vi "SeqMgr.Sequence, Parse Line.vi"(6 "Levels":cluster{"If":i32, "For":i32, "While":i32}, 8 "error in":errorcluster, 10 "LineCnt":i32, 11 "Line":string) -> (0 "error out":errorcluster, 1 "Comment":string, 2 "Is Comment":bool, 3 "Step":string[](array[string]), 4 "Levels Out":cluster{"If":i32, "For":i32, "While":i32})   [LabVIEW 2024, in "EQMF.lvlib" / "SeqMgr.lvlib"]
uses:
  SeqMgr.lvlib
  <vilib>/Utility/error.llb/Trim Whitespace One-Sided.vi
  Strings/String Utils.lvlib
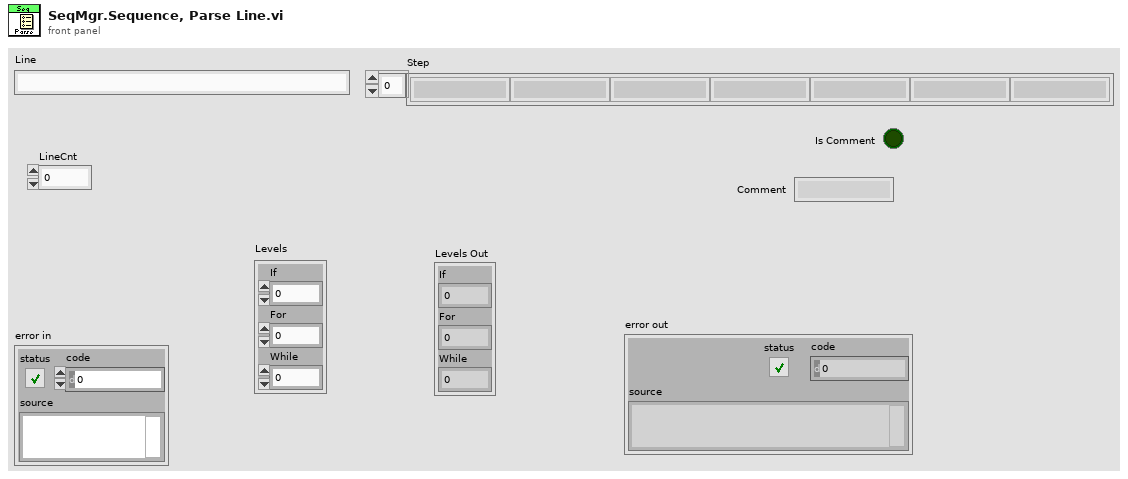
[diagram p1: front panel]
types:
  T1 = cluster{"Line":string, "Step":string[], "\nLevels":cluster{"If":i32, "For":i32, "While":i32}}
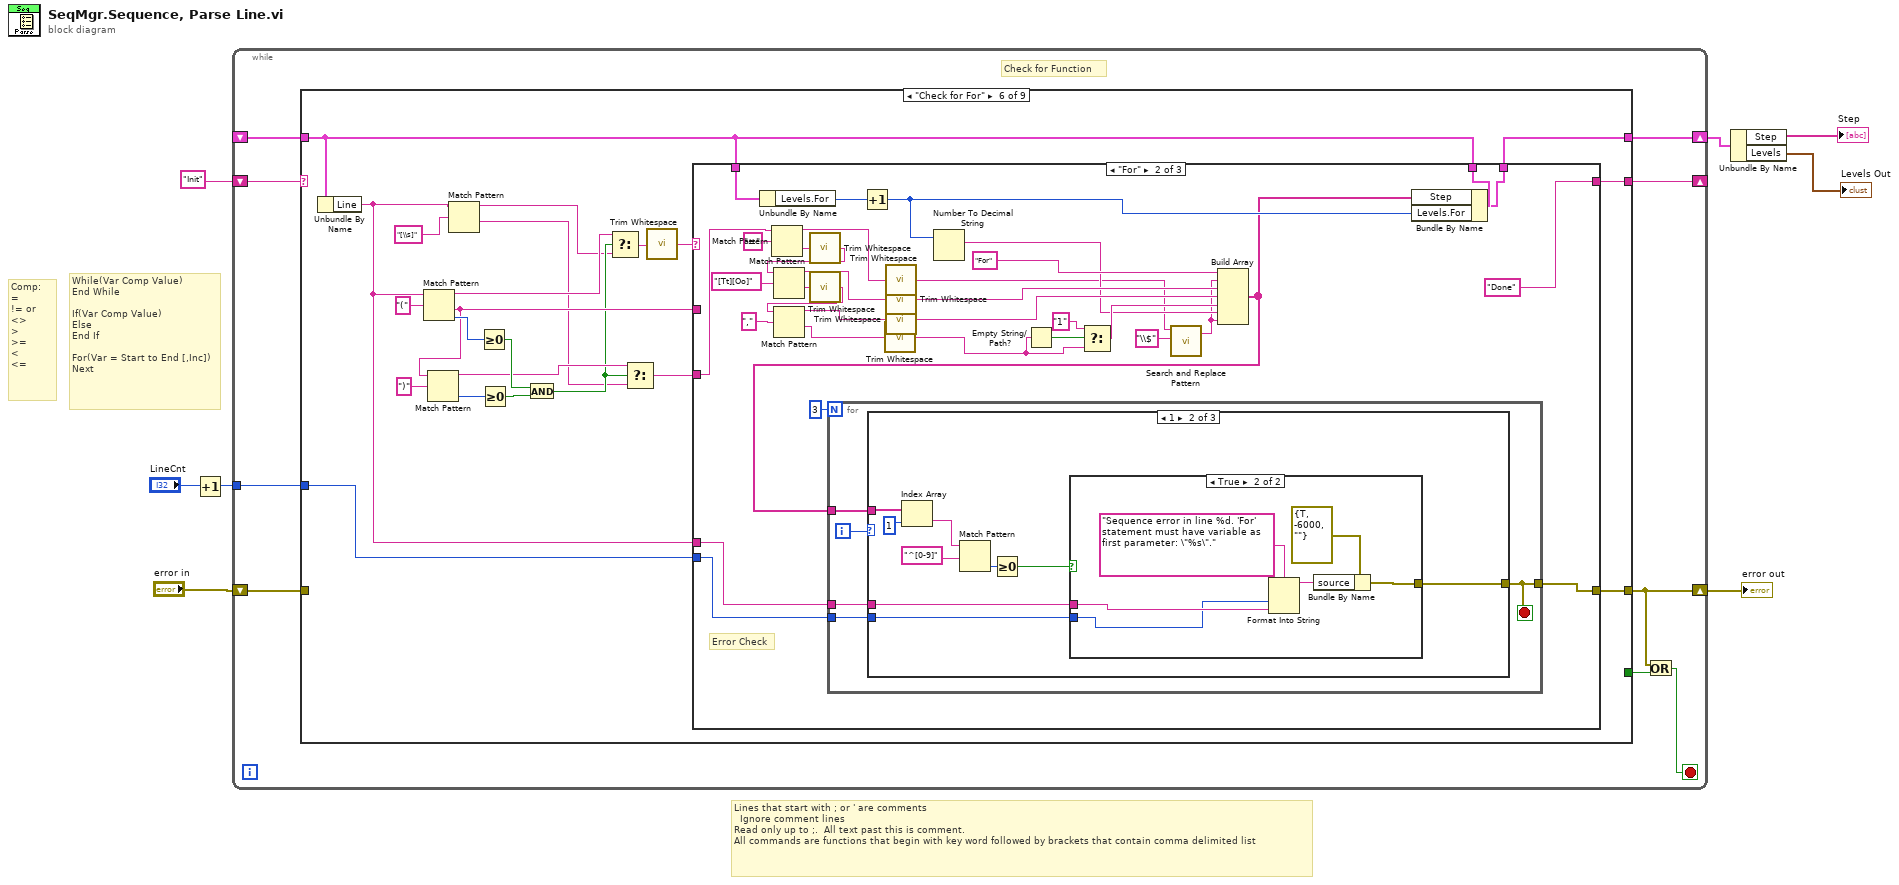
[diagram p0: block diagram]
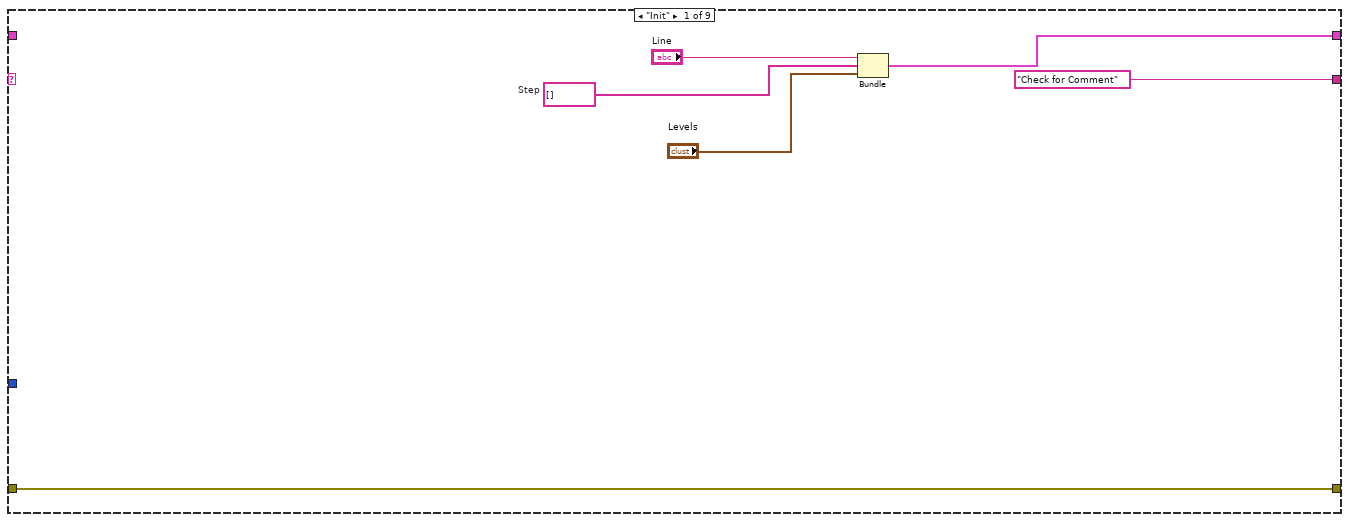
[diagram p2: hidden frame]
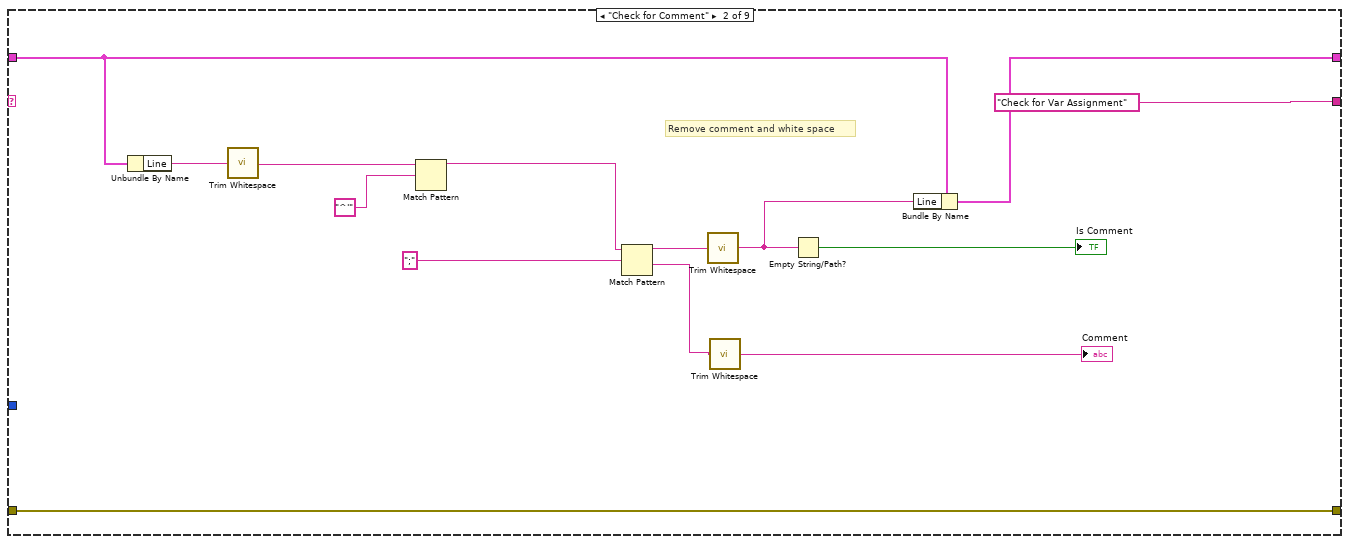
[diagram p3: hidden frame]
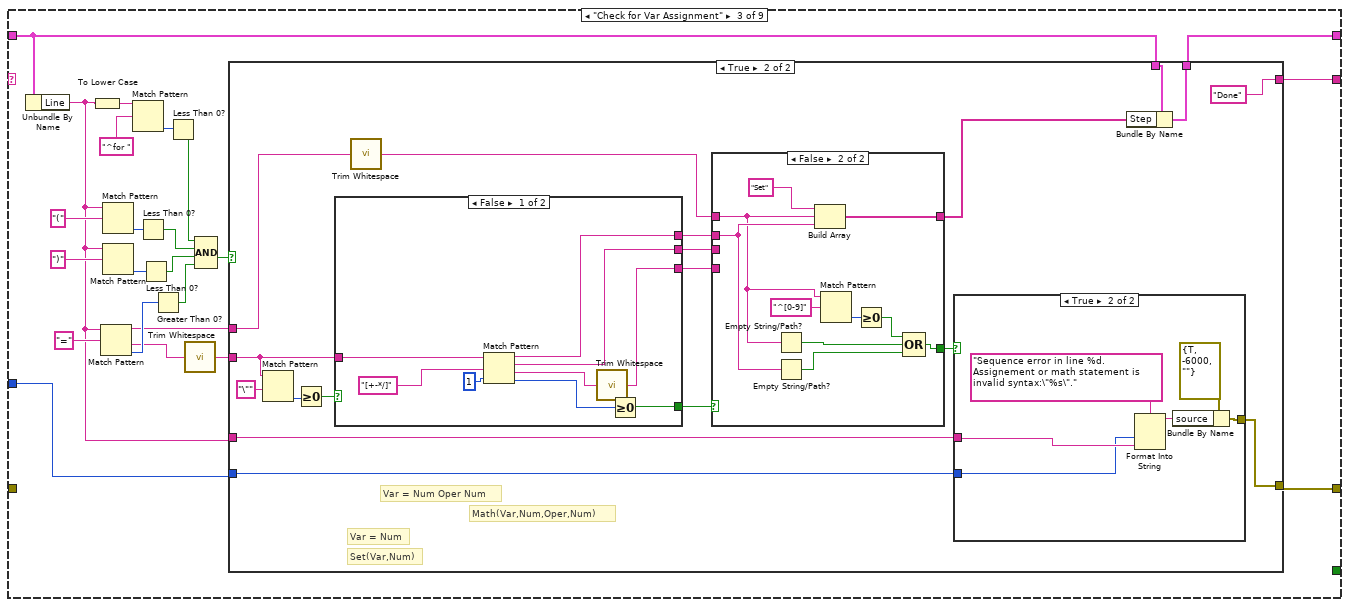
[diagram p4: hidden frame]
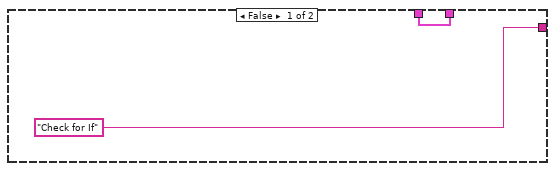
[diagram p5: hidden frame]
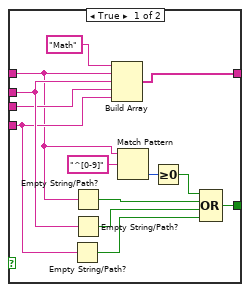
[diagram p7: hidden frame]
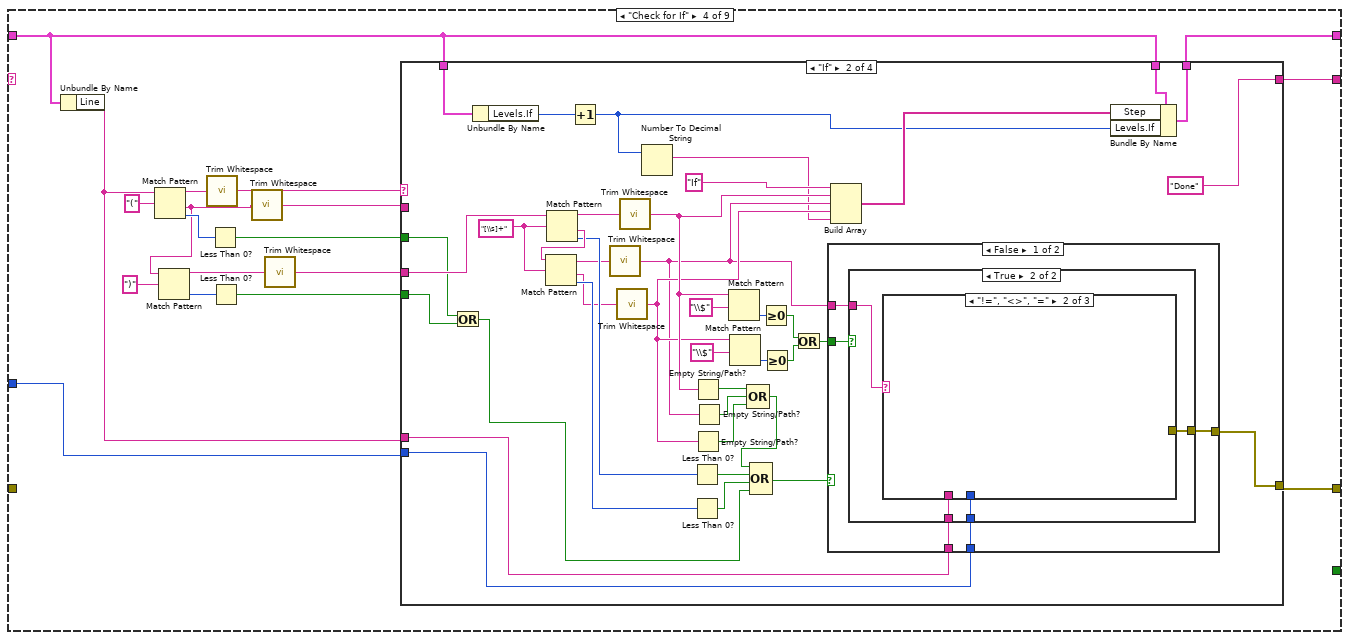
[diagram p9: hidden frame]
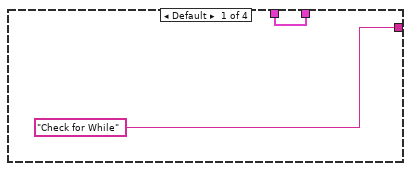
[diagram p10: hidden frame]
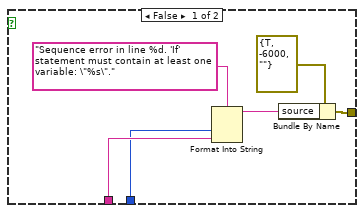
[diagram p11: hidden frame]
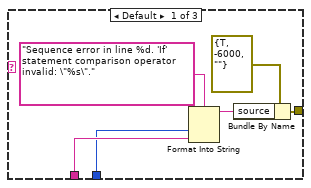
[diagram p12: hidden frame]
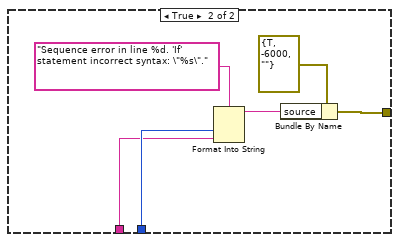
[diagram p14: hidden frame]
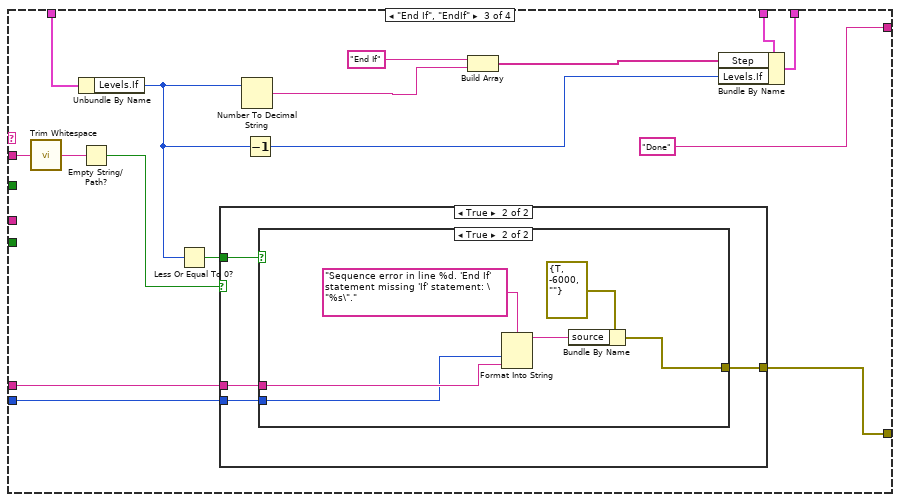
[diagram p15: hidden frame]
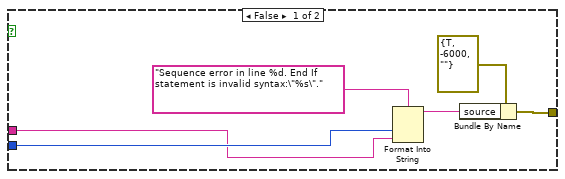
[diagram p16: hidden frame]
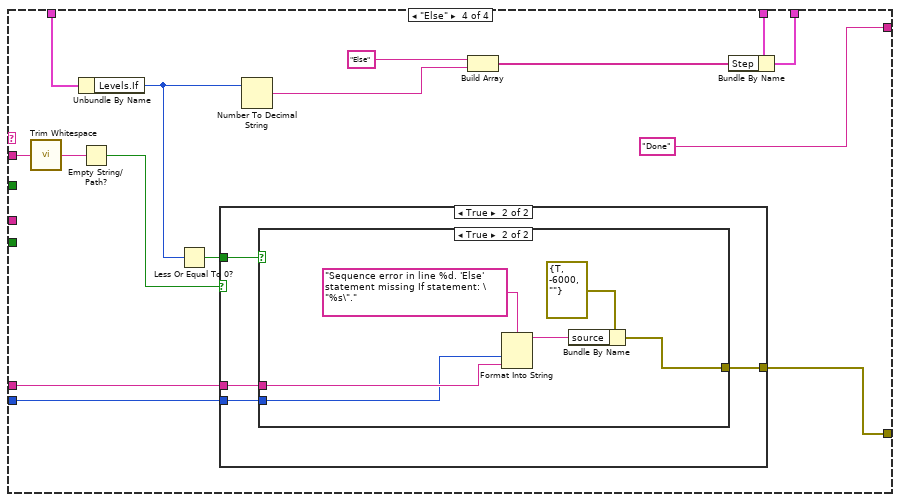
[diagram p18: hidden frame]
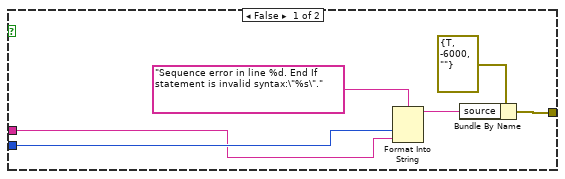
[diagram p19: hidden frame]
diagram:
  # "Comp:\n=\n!= or <>\n>\n>=\n<\n<="
  # "While(Var Comp Value)\nEnd While\n\nIf(Var Comp Value)\nElse\nEnd If\n\nFor(Var = Start to End [,Inc])\nNext"
  # "Lines that start with ; or ' are comments\n  Ignore comment lines\nRead only up to ;.  All text past this is comment.\nAll commands are functions that begin with key word followed by brackets that contain comma delimited list"
  n1 = Increment(x="LineCnt") -> (x+1=w1:i32)
  n2 = while {
    shift-right: [w11] -> _
    shift-left: "Init" -> [w17]
    shift-right: [w12] -> w5
    shift-left: _ -> [w10]
    shift-right: [w13] -> w6
    shift-left: "error in" -> [w14]
    tunnel: w1 -> [w9]
    stop <- w15 stop-if-true
    # "Check for Function"
    n3 = case shown="\"Check for For\"" w17 {
      tunnel: [_ _ _ _ _ _ _ _ TRUE] -> w16
      tunnel: w14 -> [w20 w29 _ _ _ _ _ _ w622]
      tunnel: [w20 w29 w58 w136 w284 w407 w564 w591 w622] -> w13
      tunnel: [w22 w32 w59 w137 w285 w408 w573 w604 w619] -> w12
      tunnel: ["Check for Comment" "Check for Var Assignment" w50 w135 w283 w406 "Function Error Check" "Done" _] -> w11
      tunnel: w10 -> [_ w34 w60 w131 w279 w403 w574 w604 w620]
      tunnel: w9 -> [_ _ w49 w129 w277 w402 _ _ _]
      frame "Init" {
        w23 = string[] []  # Step
        n4 = Bundle("Line"="Line", "Step"=w23, "Levels"="Levels") -> (w22:T1)  [unwired: 1 in]
      }
      frame "Check for Comment" {
        # "Remove comment and white space"
        n5 = Unbundle By Name(w34) -> ("Line"=w36:string)
        n6 = call <vilib>:"Trim Whitespace.vi"("string"=w36) -> ("trimmed string"=w26:string)  [unwired: 1 in]
        n7 = Match Pattern(string=w26, regular expression="^'") -> (before substring=w25:string)  [unwired: 1 in, 3 out]
        n8 = Match Pattern(string=w25, regular expression=";") -> (before substring=w35:string, after substring=w28:string)  [unwired: 1 in, 2 out]
        n9 = call <vilib>:"Trim Whitespace.vi"("string"=w35) -> ("trimmed string"=w33:string)  [unwired: 1 in]
        n10 = call <vilib>:"Trim Whitespace.vi"("string"=w28) -> ("trimmed string"=→"Comment":string)  [unwired: 1 in]
        n11 = Empty String/Path?(string/path=w33) -> (empty?=→"Is Comment":bool)
        n12 = Bundle By Name(cluster=w34, "Line"=w33) -> (w32:T1)
      }
      frame "Check for Var Assignment" {
        n13 = Unbundle By Name(w60) -> ("Line"=w41:string)
        n14 = To Lower Case(string=w41) -> (all lower case string=w42:string)
        n15 = Match Pattern(string=w41, regular expression="=") -> (before substring=w51:string, after substring=w43:string, offset past match=w52:i32)  [unwired: 1 in, 1 out]
        n16 = Match Pattern(string=w41, regular expression="(") -> (offset past match=w55:i32)  [unwired: 1 in, 3 out]
        n17 = Match Pattern(string=w41, regular expression=")") -> (offset past match=w54:i32)  [unwired: 1 in, 3 out]
        n18 = Match Pattern(string=w42, regular expression="^for ") -> (offset past match=w39:i32)  [unwired: 1 in, 3 out]
        n19 = Less Than 0?(x=w55) -> (x < 0?=w48:bool)
        n20 = Less Than 0?(x=w54) -> (x < 0?=w47:bool)
        n21 = Greater Than 0?(x=w52) -> (x > 0?=w46:bool)
        n22 = Less Than 0?(x=w39) -> (x < 0?=w38:bool)
        n23 = call <vilib>:"Trim Whitespace.vi"("string"=w43) -> ("trimmed string"=w44:string)  [unwired: 1 in]
        n24 = Compound Arithmetic op=AND(w38, w48, w47, w46) -> (w45:bool)
        n25 = case shown="True" w45 {
          tunnel: w60 -> [w62 w80]
          tunnel: [w62 w79] -> w59
          tunnel: [_ w78] -> w58
          tunnel: w51 -> [_ w77]
          tunnel: w44 -> [_ w66]
          tunnel: w41 -> [_ w76]
          tunnel: ["Check for If" "Done"] -> w50
          tunnel: w49 -> [_ w72]
          frame False {
          }
          frame True {
            # "Var = Num"
            # "Set(Var,Num)"
            # "Var = Num Oper Num"
            # "Math(Var,Num,Oper,Num)"
            n26 = Match Pattern(string=w66, regular expression="\"") -> (offset past match=w64:i32)  [unwired: 1 in, 3 out]
            n27 = Greater Or Equal To 0?(x=w64) -> (x >= 0?=w63:bool)
            n28 = case shown="False" w63 {
              tunnel: w66 -> [w83 w90]
              tunnel: [w87 w90] -> w71
              tunnel: [w81 _] -> w69
              tunnel: [w85 _] -> w68
              tunnel: [w84 _] -> w67
              frame False {
                n29 = Match Pattern(string=w83, regular expression="[+-*/]", offset (0)=1) -> (before substring=w87:string, match substring=w85:string, after substring=w86:string, offset past match=w89:i32)
                n30 = call <vilib>:"Trim Whitespace.vi"("string"=w86) -> ("trimmed string"=w84:string)  [unwired: 1 in]
                n31 = Greater Or Equal To 0?(x=w89) -> (x >= 0?=w81:bool)
              }
              frame True {
              }
            }
            n32 = call <vilib>:"Trim Whitespace.vi"("string"=w77) -> ("trimmed string"=w70:string)  [unwired: 1 in]
            n33 = case shown="False" w69 {
              tunnel: [w101 w111] -> w75
              tunnel: [w99 w109] -> w74
              tunnel: w71 -> [w98 w108]
              tunnel: w70 -> [w92 w105]
              tunnel: w68 -> [w97 _]
              tunnel: w67 -> [w96 _]
              frame True {
                n34 = Empty String/Path?(string/path=w96) -> (empty?=w95:bool)
                n35 = Empty String/Path?(string/path=w92) -> (empty?=w103:bool)
                n36 = Empty String/Path?(string/path=w98) -> (empty?=w102:bool)
                n37 = Build Array("Math", w92, w98, w97, w96) -> (w99:string[])
                n38 = Match Pattern(string=w92, regular expression="^[0-9]") -> (offset past match=w94:i32)  [unwired: 1 in, 3 out]
                n39 = Greater Or Equal To 0?(x=w94) -> (x >= 0?=w91:bool)
                n40 = Compound Arithmetic op=OR(w91, w103, w102, w95) -> (w101:bool)
              }
              frame False {
                n41 = Empty String/Path?(string/path=w105) -> (empty?=w113:bool)
                n42 = Empty String/Path?(string/path=w108) -> (empty?=w112:bool)
                n43 = Build Array("Set", w105, w108) -> (w109:string[])
                n44 = Match Pattern(string=w105, regular expression="^[0-9]") -> (offset past match=w107:i32)  [unwired: 1 in, 3 out]
                n45 = Greater Or Equal To 0?(x=w107) -> (x >= 0?=w104:bool)
                n46 = Compound Arithmetic op=OR(w104, w113, w112) -> (w111:bool)
              }
            }
            n47 = case shown="True" w75 {
              tunnel: w76 -> [_ w115]
              tunnel: [_ w116] -> w78
              tunnel: w72 -> [_ w114]
              frame False {
              }
              frame True {
                n48 = Format Into String(format string="Sequence error in line %d. Assignement or math statement is invalid syntax:\"%s\"." ("regular expression"), w114, w115) -> (resulting string=w117:string)  [unwired: 2 in, 1 out]
                n49 = Bundle By Name(cluster=errorcluster {"status"=TRUE, "code"=-6000, "source"=""} ("error constant"), "source"=w117) -> (w116:errorcluster)
              }
            }
            n50 = Bundle By Name(cluster=w80, "Step"=w74) -> (w79:T1)
          }
        }
      }
      frame "Check for If" {
        n51 = Unbundle By Name(w131) -> ("Line"=w130:string)
        n52 = Match Pattern(string=w130, regular expression="(") -> (before substring=w133:string, after substring=w122:string, offset past match=w128:i32)  [unwired: 1 in, 1 out]
        n53 = Match Pattern(string=w122, regular expression=")") -> (before substring=w123:string, offset past match=w125:i32)  [unwired: 1 in, 2 out]
        n54 = call <vilib>:"Trim Whitespace.vi"("string"=w133) -> ("trimmed string"=w132:string)  [unwired: 1 in]
        n55 = Less Than 0?(x=w128) -> (x < 0?=w127:bool)
        n56 = Less Than 0?(x=w125) -> (x < 0?=w124:bool)
        n57 = call <vilib>:"Trim Whitespace.vi"("string"=w122) -> ("trimmed string"=w121:string)  [unwired: 1 in]
        n58 = call <vilib>:"Trim Whitespace.vi"("string"=w123) -> ("trimmed string"=w120:string)  [unwired: 1 in]
        n59 = case shown="\"If\"" w132 {
          tunnel: w131 -> [w139 w179 w222 w253]
          tunnel: [w139 w178 w221 w252] -> w137
          tunnel: [_ w149 w220 w251] -> w136
          tunnel: w130 -> [_ w158 w219 w250]
          tunnel: ["Check for While" "Done" "Done" "Done"] -> w135
          tunnel: w121 -> [_ _ w215 w246]
          tunnel: w131 -> [_ w169 w214 w245]
          tunnel: w129 -> [_ w159 w208 w241]
          tunnel: w127 -> [_ w157 _ _]
          tunnel: w120 -> [_ w174 _ _]
          tunnel: w124 -> [_ w156 _ _]
          frame Default {
          }
          frame "If" {
            w173 = "[\\s]+"
            n60 = Or(x=w157, y=w156) -> (x .or. y?=w155:bool)
            n61 = Unbundle By Name(w169) -> ("Levels.If"=w168:i32)
            n62 = Match Pattern(string=w174, regular expression=w173) -> (before substring=w166:string, after substring=w172:string, offset past match=w171:i32)  [unwired: 1 in, 1 out]
            n63 = Match Pattern(string=w172, regular expression=w173) -> (before substring=w165:string, after substring=w140:string, offset past match=w170:i32)  [unwired: 1 in, 1 out]
            n64 = Increment(x=w168) -> (x+1=w167:i32)
            n65 = call <vilib>:"Trim Whitespace.vi"("string"=w165) -> ("trimmed string"=w142:string)  [unwired: 1 in]
            n66 = call <vilib>:"Trim Whitespace.vi"("string"=w140) -> ("trimmed string"=w145:string)  [unwired: 1 in]
            n67 = call <vilib>:"Trim Whitespace.vi"("string"=w166) -> ("trimmed string"=w152:string)  [unwired: 1 in]
            n68 = Number To Decimal String(number=w167) -> (decimal integer string=w141:string)  [unwired: 1 in]
            n69 = Less Than 0?(x=w171) -> (x < 0?=w161:bool)
            n70 = Less Than 0?(x=w170) -> (x < 0?=w160:bool)
            n71 = Empty String/Path?(string/path=w152) -> (empty?=w164:bool)
            n72 = Empty String/Path?(string/path=w145) -> (empty?=w162:bool)
            n73 = Empty String/Path?(string/path=w142) -> (empty?=w163:bool)
            n74 = Match Pattern(string=w152, regular expression="\\$") -> (offset past match=w150:i32)  [unwired: 1 in, 3 out]
            n75 = Match Pattern(string=w145, regular expression="\\$") -> (offset past match=w147:i32)  [unwired: 1 in, 3 out]
            n76 = Compound Arithmetic op=OR(w164, w163, w162) -> (w154:bool)
            n77 = Compound Arithmetic op=OR(w154, w161, w160, w155) -> (w153:bool)
            n78 = Greater Or Equal To 0?(x=w150) -> (x >= 0?=w144:bool)
            n79 = Greater Or Equal To 0?(x=w147) -> (x >= 0?=w143:bool)
            n80 = Or(x=w144, y=w143) -> (x .or. y?=w148:bool)
            n81 = case shown="False" w153 {
              tunnel: w159 -> [w182 w206]
              tunnel: w158 -> [w183 w205]
              tunnel: [w180 w201] -> w149
              tunnel: w148 -> [w184 _]
              tunnel: w142 -> [w181 _]
              frame False {
                n82 = case shown="True" w184 {
                  tunnel: w183 -> [w187 w192]
                  tunnel: w182 -> [w186 w191]
                  tunnel: w181 -> [_ w194]
                  tunnel: [w185 w193] -> w180
                  frame False {
                    n83 = Format Into String(format string="Sequence error in line %d. 'If' statement must contain at least one variable: \"%s\"." ("regular expression"), w186, w187) -> (resulting string=w190:string)  [unwired: 2 in, 1 out]
                    n84 = Bundle By Name(cluster=errorcluster {"status"=TRUE, "code"=-6000, "source"=""} ("error constant"), "source"=w190) -> (w185:errorcluster)
                  }
                  frame True {
                    n85 = case shown="\"!=\", \"<>\", \"=\"" w194 {
                      tunnel: [w197 _ _] -> w193
                      tunnel: w192 -> [w196 _ _]
                      tunnel: w191 -> [w195 _ _]
                      frame Default {
                        n86 = Format Into String(format string="Sequence error in line %d. 'If' statement comparison operator invalid: \"%s\"." ("regular expression"), w195, w196) -> (resulting string=w198:string)  [unwired: 2 in, 1 out]
                        n87 = Bundle By Name(cluster=errorcluster {"status"=TRUE, "code"=-6000, "source"=""} ("error constant"), "source"=w198) -> (w197:errorcluster)
                      }
                      frame "!=", "<>", "=" {
                      }
                      frame "<", "<=", ">", ">=" {
                      }
                    }
                  }
                }
              }
              frame True {
                n88 = Format Into String(format string="Sequence error in line %d. 'If' statement incorrect syntax: \"%s\"." ("regular expression"), w206, w205) -> (resulting string=w204:string)  [unwired: 2 in, 1 out]
                n89 = Bundle By Name(cluster=errorcluster {"status"=TRUE, "code"=-6000, "source"=""} ("error constant"), "source"=w204) -> (w201:errorcluster)
              }
            }
            n90 = Build Array("If", w152, w142, w145, w141) -> (w176:string[])
            n91 = Bundle By Name(cluster=w179, "Step"=w176, "Levels.If"=w167) -> (w178:T1)
          }
          frame "End If", "EndIf" {
            n92 = call <vilib>:"Trim Whitespace.vi"("string"=w215) -> ("trimmed string"=w213:string)  [unwired: 1 in]
            n93 = Unbundle By Name(w214) -> ("Levels.If"=w210:i32)
            n94 = Empty String/Path?(string/path=w213) -> (empty?=w212:bool)
            n95 = Less Or Equal To 0?(x=w210) -> (x <= 0?=w209:bool)
            n96 = case shown="True" w212 {
              tunnel: w219 -> [w223 w231]
              tunnel: [w225 w229] -> w220
              tunnel: w209 -> [_ w232]
              tunnel: w208 -> [w224 w230]
              frame False {
                n97 = Format Into String(format string="Sequence error in line %d. End If statement is invalid syntax:\"%s\"." ("regular expression"), w224, w223) -> (resulting string=w226:string)  [unwired: 2 in, 1 out]
                n98 = Bundle By Name(cluster=errorcluster {"status"=TRUE, "code"=-6000, "source"=""} ("error constant"), "source"=w226) -> (w225:errorcluster)
              }
              frame True {
                n99 = case shown="True" w232 {
                  tunnel: w231 -> [_ w235]
                  tunnel: w230 -> [_ w234]
                  tunnel: [_ w233] -> w229
                  frame False {
                    # "OK"
                  }
                  frame True {
                    n100 = Format Into String(format string="Sequence error in line %d. 'End If' statement missing 'If' statement: \"%s\"." ("regular expression"), w234, w235) -> (resulting string=w236:string)  [unwired: 2 in, 1 out]
                    n101 = Bundle By Name(cluster=errorcluster {"status"=TRUE, "code"=-6000, "source"=""} ("error constant"), "source"=w236) -> (w233:errorcluster)
                  }
                }
              }
            }
            n102 = Number To Decimal String(number=w210) -> (decimal integer string=w207:string)  [unwired: 1 in]
            n103 = Decrement(x=w210) -> (x-1=w211:i32)
            n104 = Build Array("End If", w207) -> (w217:string[])
            n105 = Bundle By Name(cluster=w222, "Step"=w217, "Levels.If"=w211) -> (w221:T1)
          }
          frame "Else" {
            n106 = call <vilib>:"Trim Whitespace.vi"("string"=w246) -> ("trimmed string"=w244:string)  [unwired: 1 in]
            n107 = Unbundle By Name(w245) -> ("Levels.If"=w240:i32)
            n108 = Empty String/Path?(string/path=w244) -> (empty?=w243:bool)
            n109 = Less Or Equal To 0?(x=w240) -> (x <= 0?=w242:bool)
            n110 = case shown="True" w243 {
              tunnel: w250 -> [w254 w262]
              tunnel: [w256 w260] -> w251
              tunnel: w242 -> [_ w263]
              tunnel: w241 -> [w255 w261]
              frame False {
                n111 = Format Into String(format string="Sequence error in line %d. End If statement is invalid syntax:\"%s\"." ("regular expression"), w255, w254) -> (resulting string=w257:string)  [unwired: 2 in, 1 out]
                n112 = Bundle By Name(cluster=errorcluster {"status"=TRUE, "code"=-6000, "source"=""} ("error constant"), "source"=w257) -> (w256:errorcluster)
              }
              frame True {
                n113 = case shown="True" w263 {
                  tunnel: w262 -> [_ w266]
                  tunnel: w261 -> [_ w265]
                  tunnel: [_ w264] -> w260
                  frame False {
                    # "OK"
                  }
                  frame True {
                    n114 = Format Into String(format string="Sequence error in line %d. 'Else' statement missing If statement: \"%s\"." ("regular expression"), w265, w266) -> (resulting string=w267:string)  [unwired: 2 in, 1 out]
                    n115 = Bundle By Name(cluster=errorcluster {"status"=TRUE, "code"=-6000, "source"=""} ("error constant"), "source"=w267) -> (w264:errorcluster)
                  }
                }
              }
            }
            n116 = Number To Decimal String(number=w240) -> (decimal integer string=w239:string)  [unwired: 1 in]
            n117 = Build Array("Else", w239) -> (w248:string[])
            n118 = Bundle By Name(cluster=w253, "Step"=w248) -> (w252:T1)
          }
        }
      }
      frame "Check for While" {
        n119 = Unbundle By Name(w279) -> ("Line"=w278:string)
        n120 = Match Pattern(string=w278, regular expression="(") -> (before substring=w281:string, after substring=w273:string, offset past match=w276:i32)  [unwired: 1 in, 1 out]
        n121 = Match Pattern(string=w273, regular expression=")") -> (before substring=w272:string, offset past match=w271:i32)  [unwired: 1 in, 2 out]
        n122 = call <vilib>:"Trim Whitespace.vi"("string"=w281) -> ("trimmed string"=w280:string)  [unwired: 1 in]
        n123 = Less Than 0?(x=w276) -> (x < 0?=w275:bool)
        n124 = Less Than 0?(x=w271) -> (x < 0?=w270:bool)
        n125 = case shown="\"While\"" w280 {
          tunnel: w279 -> [w287 w327 w370]
          tunnel: [w287 w326 w369] -> w285
          tunnel: [_ w297 w368] -> w284
          tunnel: w278 -> [_ w306 w367]
          tunnel: ["Check for For" "Done" "Done"] -> w283
          tunnel: w273 -> [_ _ w363]
          tunnel: w279 -> [_ w317 w362]
          tunnel: w277 -> [_ w307 w356]
          tunnel: w275 -> [_ w305 _]
          tunnel: w272 -> [_ w322 _]
          tunnel: w270 -> [_ w304 _]
          frame Default {
          }
          frame "While" {
            w321 = "[\\s]+"
            n126 = Or(x=w305, y=w304) -> (x .or. y?=w303:bool)
            n127 = Unbundle By Name(w317) -> ("Levels.While"=w316:i32)
            n128 = Match Pattern(string=w322, regular expression=w321) -> (before substring=w314:string, after substring=w320:string, offset past match=w319:i32)  [unwired: 1 in, 1 out]
            n129 = Match Pattern(string=w320, regular expression=w321) -> (before substring=w313:string, after substring=w288:string, offset past match=w318:i32)  [unwired: 1 in, 1 out]
            n130 = Increment(x=w316) -> (x+1=w315:i32)
            n131 = call <vilib>:"Trim Whitespace.vi"("string"=w313) -> ("trimmed string"=w290:string)  [unwired: 1 in]
            n132 = call <vilib>:"Trim Whitespace.vi"("string"=w288) -> ("trimmed string"=w293:string)  [unwired: 1 in]
            n133 = call <vilib>:"Trim Whitespace.vi"("string"=w314) -> ("trimmed string"=w300:string)  [unwired: 1 in]
            n134 = Number To Decimal String(number=w315) -> (decimal integer string=w289:string)  [unwired: 1 in]
            n135 = Less Than 0?(x=w319) -> (x < 0?=w309:bool)
            n136 = Less Than 0?(x=w318) -> (x < 0?=w308:bool)
            n137 = Empty String/Path?(string/path=w300) -> (empty?=w312:bool)
            n138 = Empty String/Path?(string/path=w293) -> (empty?=w310:bool)
            n139 = Empty String/Path?(string/path=w290) -> (empty?=w311:bool)
            n140 = Match Pattern(string=w300, regular expression="\\$") -> (offset past match=w298:i32)  [unwired: 1 in, 3 out]
            n141 = Match Pattern(string=w293, regular expression="\\$") -> (offset past match=w295:i32)  [unwired: 1 in, 3 out]
            n142 = Compound Arithmetic op=OR(w312, w311, w310) -> (w302:bool)
            n143 = Compound Arithmetic op=OR(w302, w309, w308, w303) -> (w301:bool)
            n144 = Greater Or Equal To 0?(x=w298) -> (x >= 0?=w292:bool)
            n145 = Greater Or Equal To 0?(x=w295) -> (x >= 0?=w291:bool)
            n146 = Or(x=w292, y=w291) -> (x .or. y?=w296:bool)
            n147 = case shown="True" w301 {
              tunnel: w307 -> [w330 w354]
              tunnel: w306 -> [w331 w353]
              tunnel: [w328 w349] -> w297
              tunnel: w296 -> [w332 _]
              tunnel: w290 -> [w329 _]
              frame False {
                n148 = case shown="False" w332 {
                  tunnel: w331 -> [w335 w340]
                  tunnel: w330 -> [w334 w339]
                  tunnel: w329 -> [_ w342]
                  tunnel: [w333 w341] -> w328
                  frame False {
                    n149 = Format Into String(format string="Sequence error in line %d. 'While' statement must contain at least one variable: \"%s\"." ("regular expression"), w334, w335) -> (resulting string=w338:string)  [unwired: 2 in, 1 out]
                    n150 = Bundle By Name(cluster=errorcluster {"status"=TRUE, "code"=-6000, "source"=""} ("error constant"), "source"=w338) -> (w333:errorcluster)
                  }
                  frame True {
                    n151 = case shown="Default" w342 {
                      tunnel: [w345 _ _] -> w341
                      tunnel: w340 -> [w344 _ _]
                      tunnel: w339 -> [w343 _ _]
                      frame Default {
                        n152 = Format Into String(format string="Sequence error in line %d. 'While' statement comparison operator invalid: \"%s\"." ("regular expression"), w343, w344) -> (resulting string=w346:string)  [unwired: 2 in, 1 out]
                        n153 = Bundle By Name(cluster=errorcluster {"status"=TRUE, "code"=-6000, "source"=""} ("error constant"), "source"=w346) -> (w345:errorcluster)
                      }
                      frame "!=", "<>", "=" {
                      }
                      frame "<", "<=", ">", ">=" {
                      }
                    }
                  }
                }
              }
              frame True {
                n154 = Format Into String(format string="Sequence error in line %d. 'While' statement incorrect syntax: \"%s\"." ("regular expression"), w354, w353) -> (resulting string=w352:string)  [unwired: 2 in, 1 out]
                n155 = Bundle By Name(cluster=errorcluster {"status"=TRUE, "code"=-6000, "source"=""} ("error constant"), "source"=w352) -> (w349:errorcluster)
              }
            }
            n156 = Build Array("While", w300, w290, w293, w289) -> (w324:string[])
            n157 = Bundle By Name(cluster=w327, "Step"=w324, "Levels.While"=w315) -> (w326:T1)
          }
          frame "End While", "EndWhile", "WEnd" {
            n158 = call <vilib>:"Trim Whitespace.vi"("string"=w363) -> ("trimmed string"=w361:string)  [unwired: 1 in]
            n159 = Unbundle By Name(w362) -> ("Levels.While"=w358:i32)
            n160 = Empty String/Path?(string/path=w361) -> (empty?=w360:bool)
            n161 = Less Or Equal To 0?(x=w358) -> (x <= 0?=w357:bool)
            n162 = case shown="False" w360 {
              tunnel: w367 -> [w371 w379]
              tunnel: [w373 w377] -> w368
              tunnel: w357 -> [_ w380]
              tunnel: w356 -> [w372 w378]
              frame False {
                n163 = Format Into String(format string="Sequence error in line %d. 'End While' statement is invalid syntax:\"%s\"." ("regular expression"), w372, w371) -> (resulting string=w374:string)  [unwired: 2 in, 1 out]
                n164 = Bundle By Name(cluster=errorcluster {"status"=TRUE, "code"=-6000, "source"=""} ("error constant"), "source"=w374) -> (w373:errorcluster)
              }
              frame True {
                n165 = case shown="True" w380 {
                  tunnel: w379 -> [_ w383]
                  tunnel: w378 -> [_ w382]
                  tunnel: [_ w381] -> w377
                  frame False {
                    # "OK"
                  }
                  frame True {
                    n166 = Format Into String(format string="Sequence error in line %d. 'End While' statement missing 'While' statement: \"%s\"." ("regular expression"), w382, w383) -> (resulting string=w384:string)  [unwired: 2 in, 1 out]
                    n167 = Bundle By Name(cluster=errorcluster {"status"=TRUE, "code"=-6000, "source"=""} ("error constant"), "source"=w384) -> (w381:errorcluster)
                  }
                }
              }
            }
            n168 = Number To Decimal String(number=w358) -> (decimal integer string=w355:string)  [unwired: 1 in]
            n169 = Decrement(x=w358) -> (x-1=w359:i32)
            n170 = Build Array("End While", w355) -> (w365:string[])
            n171 = Bundle By Name(cluster=w370, "Step"=w365, "Levels.While"=w359) -> (w369:T1)
          }
        }
      }
      frame "Check for For" {
        n172 = Unbundle By Name(w403) -> ("Line"=w387:string)
        n173 = Match Pattern(string=w387, regular expression="(") -> (before substring=w392:string, after substring=w399:string, offset past match=w401:i32)  [unwired: 1 in, 1 out]
        n174 = Match Pattern(string=w399, regular expression=")") -> (before substring=w394:string, offset past match=w398:i32)  [unwired: 1 in, 2 out]
        n175 = Match Pattern(string=w387, regular expression="[\\s]") -> (before substring=w388:string, after substring=w389:string)  [unwired: 1 in, 2 out]
        n176 = Greater Or Equal To 0?(x=w401) -> (x >= 0?=w397:bool)
        n177 = Greater Or Equal To 0?(x=w398) -> (x >= 0?=w396:bool)
        n178 = And(x=w397, y=w396) -> (x .and. y?=w390:bool)
        n179 = Select(t=w392, s=w390, f=w388) -> (s? t:f=w391:string)
        n180 = Select(t=w394, s=w390, f=w389) -> (s? t:f=w393:string)
        n181 = call <vilib>:"Trim Whitespace.vi"("string"=w391) -> ("trimmed string"=w404:string)  [unwired: 1 in]
        n182 = case shown="\"For\"" w404 {
          tunnel: w403 -> [w410 w444 w541]
          tunnel: [w410 w443 w540] -> w408
          tunnel: [_ w428 w539] -> w407
          tunnel: w387 -> [_ w431 w538]
          tunnel: ["Check for Function" "Done" "Done"] -> w406
          tunnel: w399 -> [_ _ w534]
          tunnel: w403 -> [_ w440 w533]
          tunnel: w402 -> [_ w430 w527]
          tunnel: w393 -> [_ w412 _]
          frame Default {
          }
          frame "For" {
            # "Error Check"
            n183 = Unbundle By Name(w440) -> ("Levels.For"=w439:i32)
            n184 = Match Pattern(string=w412, regular expression="=") -> (before substring=w421:string, after substring=w419:string)  [unwired: 1 in, 2 out]
            n185 = call <vilib>:"Trim Whitespace.vi"("string"=w419) -> ("trimmed string"=w418:string)  [unwired: 1 in]
            n186 = Match Pattern(string=w418, regular expression="[Tt][Oo]") -> (before substring=w420:string, after substring=w417:string)  [unwired: 1 in, 2 out]
            n187 = call <vilib>:"Trim Whitespace.vi"("string"=w417) -> ("trimmed string"=w416:string)  [unwired: 1 in]
            n188 = Match Pattern(string=w416, regular expression=",") -> (before substring=w414:string, after substring=w413:string)  [unwired: 1 in, 2 out]
            n189 = Increment(x=w439) -> (x+1=w438:i32)
            n190 = call <vilib>:"Trim Whitespace.vi"("string"=w413) -> ("trimmed string"=w433:string)  [unwired: 1 in]
            n191 = call <vilib>:"Trim Whitespace.vi"("string"=w421) -> ("trimmed string"=w426:string)  [unwired: 1 in]
            n192 = call <vilib>:"Trim Whitespace.vi"("string"=w420) -> ("trimmed string"=w437:string)  [unwired: 1 in]
            n193 = call <vilib>:"Trim Whitespace.vi"("string"=w414) -> ("trimmed string"=w436:string)  [unwired: 1 in]
            n194 = Number To Decimal String(number=w438) -> (decimal integer string=w427:string)  [unwired: 1 in]
            n195 = Empty String/Path?(string/path=w433) -> (empty?=w435:bool)
            n196 = Select(t="1", s=w435, f=w433) -> (s? t:f=w432:string)
            n197 = call <vilib>:"Search and Replace Pattern.vi"("string"=w426, "regular expression (\"\")"="\\$") -> ("result string"=w424:string)  [unwired: 3 in, 1 out]
            n198 = Build Array("For", w424, w437, w436, w432, w427, w424) -> (w429:string[])
            n199 = for {
              N: 3 -> [_]
              tunnel: w431 -> [w448]
              tunnel: w430 -> [w447]
              tunnel: w429 -> [w446]
              tunnel: [w445] -> w428
              i -> [w449]
              stop <- w445 stop-if-true
              n200 = case shown="1" w449 {
                tunnel: w448 -> [w452 w474 w499]
                tunnel: w447 -> [w451 w473 w498]
                tunnel: w446 -> [w461 w476 w493]
                tunnel: [w450 w472 w497] -> w445
                frame 0, Default {
                  n201 = Index Array(array=w461, index #1=1 ("index")) -> (element #1=w460:string, element #2=w459:string, element #3=w458:string)  [unwired: 2 in]
                  n202 = Empty String/Path?(string/path=w460) -> (empty?=w456:bool)
                  n203 = Empty String/Path?(string/path=w459) -> (empty?=w455:bool)
                  n204 = Empty String/Path?(string/path=w458) -> (empty?=w454:bool)
                  n205 = Compound Arithmetic op=OR(w456, w455, w454) -> (w453:bool)
                  n206 = case shown="True" w453 {
                    tunnel: w452 -> [_ w464]
                    tunnel: w451 -> [_ w463]
                    tunnel: [_ w462] -> w450
                    frame False {
                    }
                    frame True {
                      n207 = Format Into String(format string="Sequence error in line %d. 'For' statement missing a parameter: \"%s\"." ("regular expression"), w463, w464) -> (resulting string=w465:string)  [unwired: 2 in, 1 out]
                      n208 = Bundle By Name(cluster=errorcluster {"status"=TRUE, "code"=-6000, "source"=""} ("error constant"), "source"=w465) -> (w462:errorcluster)
                    }
                  }
                }
                frame 1 {
                  n209 = Index Array(array=w476, index=1) -> (element=w469:string)
                  n210 = Match Pattern(string=w469, regular expression="^[0-9]") -> (offset past match=w470:i32)  [unwired: 1 in, 3 out]
                  n211 = Greater Or Equal To 0?(x=w470) -> (x >= 0?=w468:bool)
                  n212 = case shown="True" w468 {
                    tunnel: w474 -> [_ w479]
                    tunnel: w473 -> [_ w478]
                    tunnel: [_ w477] -> w472
                    frame False {
                    }
                    frame True {
                      n213 = Format Into String(format string="Sequence error in line %d. 'For' statement must have variable as first parameter: \"%s\"." ("regular expression"), w478, w479) -> (resulting string=w480:string)  [unwired: 2 in, 1 out]
                      n214 = Bundle By Name(cluster=errorcluster {"status"=TRUE, "code"=-6000, "source"=""} ("error constant"), "source"=w480) -> (w477:errorcluster)
                    }
                  }
                }
                frame 2 {
                  w491 = "%f"
                  # "Need to ignore if are vars"
                  n215 = Index Array(array=w493, index #1=2 ("index")) -> (element #1=w495:string, element #2=w494:string, element #3=w492:string)  [unwired: 2 in]
                  n216 = Scan From String(format string=w491, input string=w492) -> (error out=w488:errorcluster, output 1=w486:dbl)  [unwired: 3 in, 2 out]
                  n217 = Scan From String(format string=w491, input string=w494) -> (error out=w489:errorcluster, output 1=w485:dbl)  [unwired: 3 in, 2 out]
                  n218 = Scan From String(format string=w491, input string=w495) -> (error out=w490:errorcluster, output 1=w487:dbl)  [unwired: 3 in, 2 out]
                  n219 = Merge Errors(w490, w489, w488) -> (w483:errorcluster)
                  n220 = case shown="False" FALSE {
                    selector: FALSE -> [w500 _]
                    tunnel: w499 -> [w503 w512]
                    tunnel: w498 -> [w502 w511]
                    tunnel: [w501 w513] -> w497
                    tunnel: w487 -> [_ w518]
                    tunnel: w486 -> [_ w519]
                    tunnel: w485 -> [_ w517]
                    tunnel: w483 -> [_ _]
                    frame False {
                      n221 = case shown="False" w500 {
                        tunnel: w503 -> [_ w506]
                        tunnel: w502 -> [_ w505]
                        tunnel: [_ w504] -> w501
                        frame False {
                        }
                        frame True {
                          n222 = Format Into String(format string="Sequence error in line %d. 'For' statement must have numeric Start, End, and Inc parameters: \"%s\"." ("regular expression"), w505, w506) -> (resulting string=w507:string)  [unwired: 2 in, 1 out]
                          n223 = Bundle By Name(cluster=errorcluster {"status"=TRUE, "code"=-6000, "source"=""} ("error constant"), "source"=w507) -> (w504:errorcluster)
                        }
                      }
                    }
                    frame True {
                      n224 = Greater Than 0?(x=w519) -> (x > 0?=w514:bool)
                      n225 = Less?(x=w518, y=w517) -> (x < y?=w516:bool)
                      n226 = Greater?(x=w518, y=w517) -> (0:w515:bool)
                      n227 = Select(t=w516, s=w514, f=w515) -> (s? t:f=w510:bool)
                      n228 = case shown="True" w510 {
                        tunnel: [_ w522] -> w513
                        tunnel: w512 -> [_ w521]
                        tunnel: w511 -> [_ w520]
                        frame False {
                        }
                        frame True {
                          n229 = Format Into String(format string="Sequence error in line %d. 'For' statement has incorrect Start, End and Inc params (: \"%s\"." ("regular expression"), w520, w521) -> (resulting string=w523:string)  [unwired: 2 in, 1 out]
                          n230 = Bundle By Name(cluster=errorcluster {"status"=TRUE, "code"=-6000, "source"=""} ("error constant"), "source"=w523) -> (w522:errorcluster)
                        }
                      }
                    }
                  }
                }
              }
            }
            n231 = Bundle By Name(cluster=w444, "Step"=w429, "Levels.For"=w438) -> (w443:T1)
          }
          frame "Next" {
            n232 = call <vilib>:"Trim Whitespace.vi"("string"=w534) -> ("trimmed string"=w532:string)  [unwired: 1 in]
            n233 = Unbundle By Name(w533) -> ("Levels.For"=w529:i32)
            n234 = Empty String/Path?(string/path=w532) -> (empty?=w531:bool)
            n235 = Less Or Equal To 0?(x=w529) -> (x <= 0?=w528:bool)
            n236 = case shown="True" w531 {
              tunnel: w538 -> [w542 w550]
              tunnel: [w544 w548] -> w539
              tunnel: w528 -> [_ w551]
              tunnel: w527 -> [w543 w549]
              frame False {
                n237 = Format Into String(format string="Sequence error in line %d. 'Next' statement is invalid syntax:\"%s\"." ("regular expression"), w543, w542) -> (resulting string=w545:string)  [unwired: 2 in, 1 out]
                n238 = Bundle By Name(cluster=errorcluster {"status"=TRUE, "code"=-6000, "source"=""} ("error constant"), "source"=w545) -> (w544:errorcluster)
              }
              frame True {
                n239 = case shown="True" w551 {
                  tunnel: w550 -> [_ w554]
                  tunnel: w549 -> [_ w553]
                  tunnel: [_ w552] -> w548
                  frame False {
                    # "OK"
                  }
                  frame True {
                    n240 = Format Into String(format string="Sequence error in line %d. 'Next' statement missing 'For' statement: \"%s\"." ("regular expression"), w553, w554) -> (resulting string=w555:string)  [unwired: 2 in, 1 out]
                    n241 = Bundle By Name(cluster=errorcluster {"status"=TRUE, "code"=-6000, "source"=""} ("error constant"), "source"=w555) -> (w552:errorcluster)
                  }
                }
              }
            }
            n242 = Number To Decimal String(number=w529) -> (decimal integer string=w526:string)  [unwired: 1 in]
            n243 = Decrement(x=w529) -> (x-1=w530:i32)
            n244 = Build Array("Next", w526) -> (w536:string[])
            n245 = Bundle By Name(cluster=w541, "Step"=w536, "Levels.For"=w530) -> (w540:T1)
          }
        }
      }
      frame "Check for Function" {
        n246 = Unbundle By Name(w574) -> ("Line"=w562:string)
        n247 = Match Pattern(string=w562, regular expression="(") -> (before substring=w568:string, after substring=w576:string, offset past match=w571:i32)  [unwired: 1 in, 1 out]
        n248 = Match Pattern(string=w576, regular expression=")") -> (before substring=w560:string)  [unwired: 1 in, 3 out]
        n249 = Match Pattern(string=w562, regular expression=")") -> (offset past match=w561:i32)  [unwired: 1 in, 3 out]
        n250 = call <vilib>:"Trim Whitespace.vi"("string"=w568) -> ("trimmed string"=w567:string)  [unwired: 1 in]
        n251 = Less Than 0?(x=w561) -> (x < 0?=w569:bool)
        n252 = Less Than 0?(x=w571) -> (x < 0?=w570:bool)
        n253 = Exclusive Or(1:w569, 2:w570) -> (0:w565:bool)
        n254 = call "String.Convert CSV Line with Quotes to 1D Array.vi"("CSV String"=w560) -> ("Array"=w559:string[])  [unwired: 9 in, 1 out]
        n255 = case shown="False" FALSE {
          tunnel: [w579 w581] -> w575
          tunnel: w567 -> [w579 w580]
          frame False {
          }
          frame True {
            n256 = To Lower Case(string=w580) -> (all lower case string=w581:string)
          }
        }
        n257 = case shown="False" w565 {
          tunnel: w562 -> [_ w586]
          tunnel: [_ w583] -> w564
          tunnel: w561 -> [_ w582]
          frame False {
          }
          frame True {
            n258 = case shown="0, Default" w582 {
              tunnel: ["Sequence file function missing left bracket:\"%s\"." ("regular expression") "Sequence file function missing right bracket:\"%s\"." ("regular expression")] -> w587
              frame 0, Default {
              }
              frame -1 {
              }
            }
            n259 = Format Into String(format string=w587, w586) -> (resulting string=w584:string)  [unwired: 2 in, 1 out]
            n260 = Bundle By Name(cluster=errorcluster {"status"=TRUE, "code"=-6000, "source"=""} ("error constant"), "source"=w584) -> (w583:errorcluster)
          }
        }
        n261 = Build Array (concatenate)(w575, w559) -> (w572:string[])
        n262 = Bundle By Name(cluster=w574, "Step"=w572) -> (w573:T1)
      }
      frame "Function Error Check" {
        n263 = Unbundle By Name(w604) -> ("Line"=w603:string, "Step"=w602:string[])
        n264 = Delete From Array(array=w602, length=1, index=0) -> (deleted portion=w598:string[], array with subset deleted=w601:string[])
        n265 = Index Array(array=w598) -> (element=w596:string)  [unwired: 1 in]
        n266 = for {
          tunnel: w601 -> [w608] mode=indexing
          tunnel: "[()]" ("regular expression") -> [w607]
          tunnel: [w606] -> w592
          stop <- w606 stop-if-true
          n267 = Match Pattern(string=w608, regular expression=w607) -> (offset past match=w609:i32)  [unwired: 1 in, 3 out]
          n268 = Greater Or Equal To 0?(x=w609) -> (x >= 0?=w606:bool)
        }
        n269 = Match Pattern(string=w596, regular expression="[()\\s,]") -> (offset past match=w597:i32)  [unwired: 1 in, 3 out]
        n270 = Greater Or Equal To 0?(x=w597) -> (x >= 0?=w594:bool)
        n271 = Or(x=w592, y=w594) -> (x .or. y?=w593:bool)
        n272 = case shown="False" w593 {
          tunnel: w603 -> [_ w614]
          tunnel: [_ w611] -> w591
          tunnel: w592 -> [_ w610]
          frame False {
          }
          frame True {
            n273 = case shown="True" w610 {
              tunnel: ["Sequence file function parameter contains invalid character(s): \"%s\"." ("regular expression") "Function name contains illegal character(s) or is missing brackets: \"%s\"." ("regular expression")] -> w615
              frame True {
              }
              frame False {
              }
            }
            n274 = Format Into String(format string=w615, w614) -> (resulting string=w612:string)  [unwired: 2 in, 1 out]
            n275 = Bundle By Name(cluster=errorcluster {"status"=TRUE, "code"=-5000, "source"=""} ("error constant"), "source"=w612) -> (w611:errorcluster)
          }
        }
      }
      frame "Done", Default {
        n276 = Unbundle By Name(w620) -> ("Step"=w621:string[])
        n277 = for {
          tunnel: w621 -> [w625] mode=indexing
          tunnel: [w624] -> w618 mode=indexing
          n278 = call "String.Remove Start and End Quotes.vi"("String In"=w625) -> ("String Out"=w624:string)  [unwired: 9 in, 1 out]
        }
        n279 = Bundle By Name(cluster=w620, "Step"=w618) -> (w619:T1)
      }
    }
    n280 = Or(x=w13, y=w16) -> (x .or. y?=w15:bool)
  }
  "error out" <- w6
  n281 = Unbundle By Name(w5) -> ("Step"=→"Step":string[], "Levels"=→"Levels Out":cluster{"If":i32, "For":i32, "While":i32})
